vi "Send and read from TCP Server.vi"(6 "timeout (ms)":i32=1000, 8 "error in (no error)":errorcluster, 10 "Message":string, 11 "GD ID":string) -> (0 "error out":errorcluster, 3 "Reply":string)   [LabVIEW 2026, in "TALOS.lvlib"]
uses:
  TALOS.lvlib
  Ancestor/Ancestor/Ancestor.lvclass/Ancestor.ctl
  Generate Error.vi
  FGV/Error Memory/Get Error Description.vi
  Get PC name.vi
  Ancestor/Ancestor/Read ID.vi
  Get Class Name.vi
  <vilib>/Utility/error.llb/Clear Errors.vi
  FGV/Error Memory/Error Memory Core.vi
  <vilib>/AdvancedString/Delimited String to 1D String Array.vi
  <vilib>/AdvancedString/Delimited String to 1D String Array (string).vi
  Circus Root Path.vi
  FGV/Error Memory/Error Crt Lvl checker.vi
  FGV/Error Memory/Error Memory Core.vi/40c8088d-b597-4017-91af-faa98e00292e.vi
  FGV/Error Memory/Error Memory Core.vi/d4a3ab98-063c-4e44-b43d-fbdcfe6c2be2.vi
  Global Memory.vi
  <vilib>/Utility/LVClass/Get LV Class Name.vi
  Is in Packed Library.vi
  TALOS Root path.vi
  Read CSV worksheet.vi
  Global Constants.vi
  <vilib>/Utility/error.llb/General Error Handler.vi
  Error Log.vi
  Ancestor/Ancestor/Ancestor.lvclass
  <vilib>/Comparison/Equal/Equal Functor/Equal Functor.lvclass
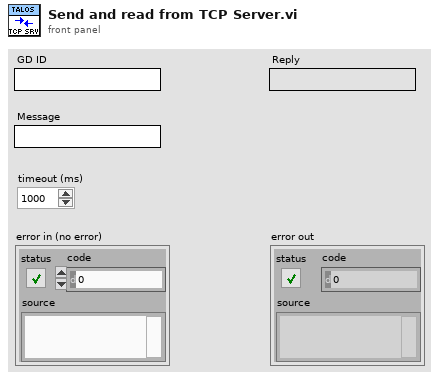
[diagram p1: front panel]
types:
  T1 = enum16{"Standard", "Buffered", "CRLF", "Immediate"}
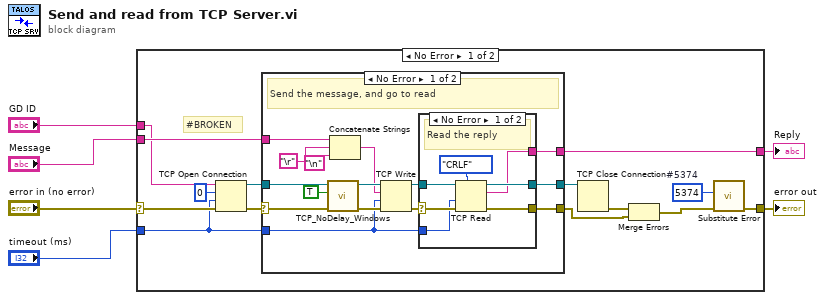
[diagram p0: block diagram]
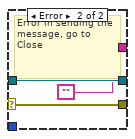
[diagram p2: hidden frame]
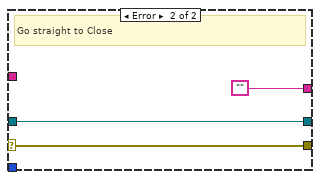
[diagram p3: hidden frame]
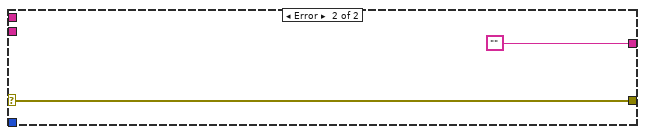
[diagram p4: hidden frame]
diagram:
  n1 = case shown="No Error" "error in (no error)" {
    selector: "error in (no error)" -> [w15 w50]
    tunnel: "Message" -> [w16 _]
    tunnel: "GD ID" -> [w8 _]
    tunnel: [w12 w50] -> w3
    tunnel: [w10 ""] -> w2
    tunnel: "timeout (ms)" -> [w9 _]
    frame No Error {
      w11 = 5374  # #5374
      # "#BROKEN"
      n2 = TCP Open Connection(address=w8, remote port or service name=u16 0, timeout ms (60000)=w9, error in (no error)=w15) -> (connection ID=w17:refnum<k5>, error out=w18:errorcluster)  [unwired: 1 in]
      n3 = case shown="No Error" w18 {
        selector: w18 -> [w35 w48]
        tunnel: w9 -> [w24 _]
        tunnel: [w23 w47] -> w19
        tunnel: w17 -> [w32 w47]
        tunnel: w16 -> [w27 _]
        tunnel: [w22 w48] -> w14
        tunnel: [w21 ""] -> w10
        frame No Error {
          # "Send the message, and go to read"
          n4 = call "TCP_NoDelay_Windows.vi"("error in (no error)"=w35, "TCP_NODELAY (true)"=TRUE, "connID"=w32) -> ("error out"=w34:errorcluster, "connID 2"=w33:refnum<k5>)  [unwired: 3 in]
          n5 = Concatenate Strings(w27, "\r", "\n") -> (w28:string)
          n6 = TCP Write(connection ID=w33, data in=w28, error in (no error)=w34, 9:w24) -> (connection ID out=w25:refnum<k5>, error out=w26:errorcluster)  [unwired: 1 out]
          n7 = case shown="No Error" w26 {
            selector: w26 -> [w41 w44]
            tunnel: w25 -> [w42 w45]
            tunnel: w24 -> [w40 _]
            tunnel: [w38 w45] -> w23
            tunnel: [w37 w44] -> w22
            tunnel: [w36 ""] -> w21
            frame No Error {
              # "Read the reply"
              n8 = TCP Read(connection ID=w42, error in (no error)=w41, 7:T1."CRLF" ("mode (standard)"), 9:w40) -> (connection ID out=w38:refnum<k5>, data out=w36:string, error out=w37:errorcluster)  [unwired: 1 in]
            }
            frame Error {
              # "Error in sending the message, go to Close"
            }
          }
        }
        frame Error {
          # "Go straight to Close"
        }
      }
      n9 = TCP Close Connection(connection ID=w19) -> (error out=w20:errorcluster)  [unwired: 2 in, 1 out]
      n10 = Merge Errors(w20, w14) -> (w13:errorcluster)
      n11 = call "Substitute Error.vi"("error in (no error)"=w13, "Error Code"=w11) -> ("error out"=w12:errorcluster)  [unwired: 9 in]
    }
    frame Error {
    }
  }
  "error out" <- w3
  "Reply" <- w2
